vi "WriteCustomError.vi"(1 "Source":string, 2 "Code":u32) -> (0 "error out":errorcluster)   [LabVIEW 2016]
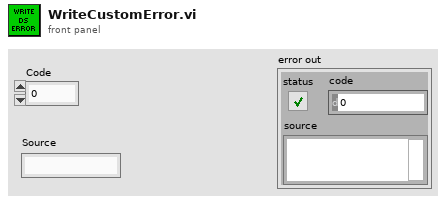
[diagram p1: front panel]
types:
  T1 = cluster{"Status":bool, "Code":u32, "Source":string}
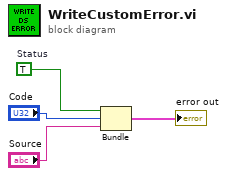
[diagram p0: block diagram]
diagram:
  w4 = TRUE  # Status
  n1 = Bundle("Status"=w4, "Code"="Code", "Source"="Source") -> (→"error out":T1)  [unwired: 1 in]
